vi "Get Image.vi"(8 "error in (no error)":errorcluster, 9 "Reset Stats?":bool, 10 "Calc Stats?":bool, 11 "ICamera in":refnum<class "ICamera.lvclass">) -> (0 "error out":errorcluster, 2 "Image out":T1, 3 "ICamera out":refnum<class "ICamera.lvclass">)   [LabVIEW 2023, in "HAL Interfaces.lvlib" / "ICamera.lvclass"]
uses:
  ICamera.lvclass
  <vilib>/vision/Image Controls.llb/IMAQ Image.ctl
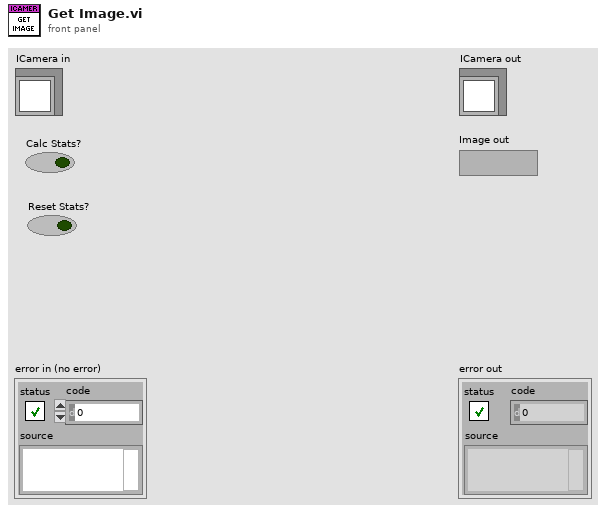
[diagram p1: front panel]
types:
  T1 = typedef "IMAQ Image.ctl" = refnum<image>
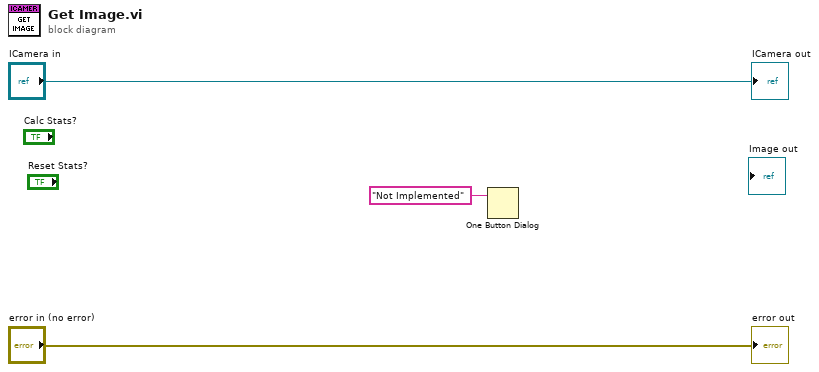
[diagram p0: block diagram]
diagram:
  n1 = One Button Dialog(message="Not Implemented") -> ()  [unwired: 1 in, 1 out]
  "error out" <- "error in (no error)"
  "ICamera out" <- "ICamera in"
